vi "buildTerminalName.vi"(8 "error in (no error)":errorcluster, 9 "Local Terminal Name":string, 10 "Channel Name":string, 11 "session handle":refnum<k15>) -> (0 "error IO":errorcluster, 2 "Fully Qualified Terminal Name":string, 3 "session handle 2":refnum<k15>)   [LabVIEW 2021]
doc: "This SubVI builds a fully qualified terminal name (such as \"/dev1/Engine0/StartTrigger\") based off of the device name, desired channel and desired local terminal name."
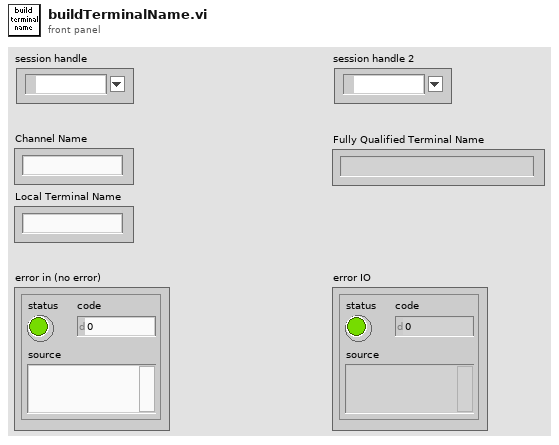
[diagram p1: front panel]
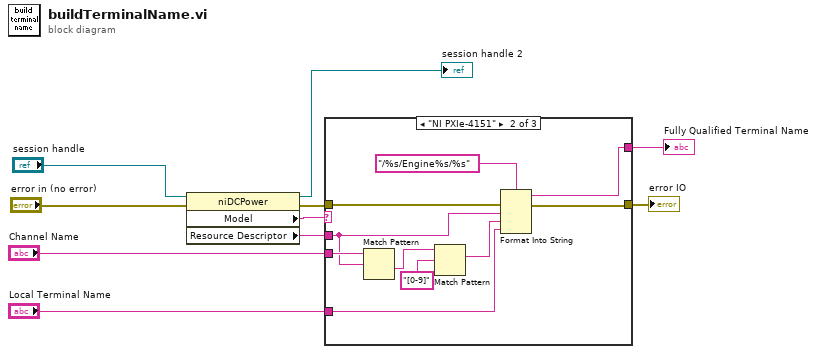
[diagram p0: block diagram]
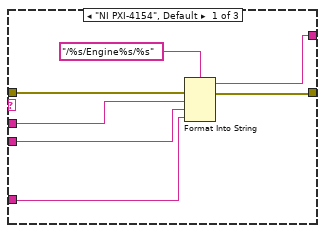
[diagram p2: hidden frame]
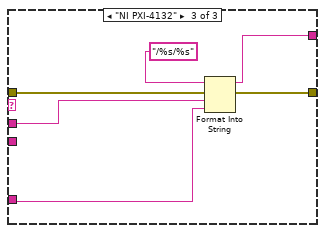
[diagram p3: hidden frame]
diagram:
  n1 = property class="niDCPower"(reference="session handle", error in="error in (no error)") -> (reference out=→"session handle 2":refnum<k15>, error out=w6:errorcluster, "Model"=w10:string, "Resource Descriptor"=w2:string)
  n2 = case shown="\"NI PXIe-4151\"" w10 {
    tunnel: w6 -> [w17 w27 w33]
    tunnel: [w16 w26 w32] -> w5
    tunnel: [w15 w25 w31] -> w4
    tunnel: "Local Terminal Name" -> [w13 w23 w29]
    tunnel: w2 -> [w12 w19 w28]
    tunnel: "Channel Name" -> [w11 w20 _]
    frame "NI PXI-4154", Default {
      n3 = Format Into String(format string="/%s/Engine%s/%s", error in=w17, w12, w11, w13) -> (resulting string=w15:string, error out=w16:errorcluster)  [unwired: 1 in]
    }
    frame "NI PXIe-4151" {
      n4 = Match Pattern(string=w20, regular expression=w19) -> (after substring=w18:string)  [unwired: 1 in, 3 out]
      n5 = Match Pattern(string=w18, regular expression="[0-9]") -> (match substring=w22:string)  [unwired: 1 in, 3 out]
      n6 = Format Into String(format string="/%s/Engine%s/%s", error in=w27, w19, w22, w23) -> (resulting string=w25:string, error out=w26:errorcluster)  [unwired: 1 in]
    }
    frame "NI PXI-4132" {
      n7 = Format Into String(format string="/%s/%s", error in=w33, w28, w29) -> (resulting string=w31:string, error out=w32:errorcluster)  [unwired: 1 in]
    }
  }
  "error IO" <- w5
  "Fully Qualified Terminal Name" <- w4
